vi "纳清DO电极校准.vi"() -> ()   [LabVIEW 2016, in "斯坦道多参数.lvlib"]
uses:
  <vilib>/Utility/miscctls.llb/LVPointTypeDef.ctl
  <vilib>/Analysis/NI_AALBase.lvlib
panel:
  out "滤波设定":dbl
  out "标液2":string="饱和标准液"
  out "标液1":string="零点标准液"
  out "第二点信号值":dbl
  out "第一点信号值":dbl
  out "盐度":sgl format="%#.2f"
  out "大气压力":dbl format="%#.2f"
  out "饱和值":sgl format="%#.2f"
  out "报警信息":string
  out "通讯状态":string
  out "第二点校准值":dbl
  out "第一点校准值":dbl
  in  "校准停止":bool
  in  "校准启动":bool
  in  "校准模式":u16(ring)=1 items=["两点校准", "单点校准"]
  out "最小值":sgl format="%#.2f"
  out "最大值":sgl format="%#.2f"
  out "波形图表":dbl(graph) caption="历史曲线"
  out "mean":dbl caption="均值" format="%#.2f"
  out "standard deviation":dbl caption="标准差" format="%#.2f"
  out "变异系数":dbl format="%#.6f"
  out "测量值":sgl format="%#.2f"
  out "提示":string
  out "原始光强数值":sgl caption="信号值" format="%#.6f"
  out "温度":dbl format="%#.2f"
  # "DO电极设定"
  # "℃"
  # "mg/L"
  # "%"
  # "nA"
  # "kPa"
  # "ppt"
  # "请选择校准模式:"
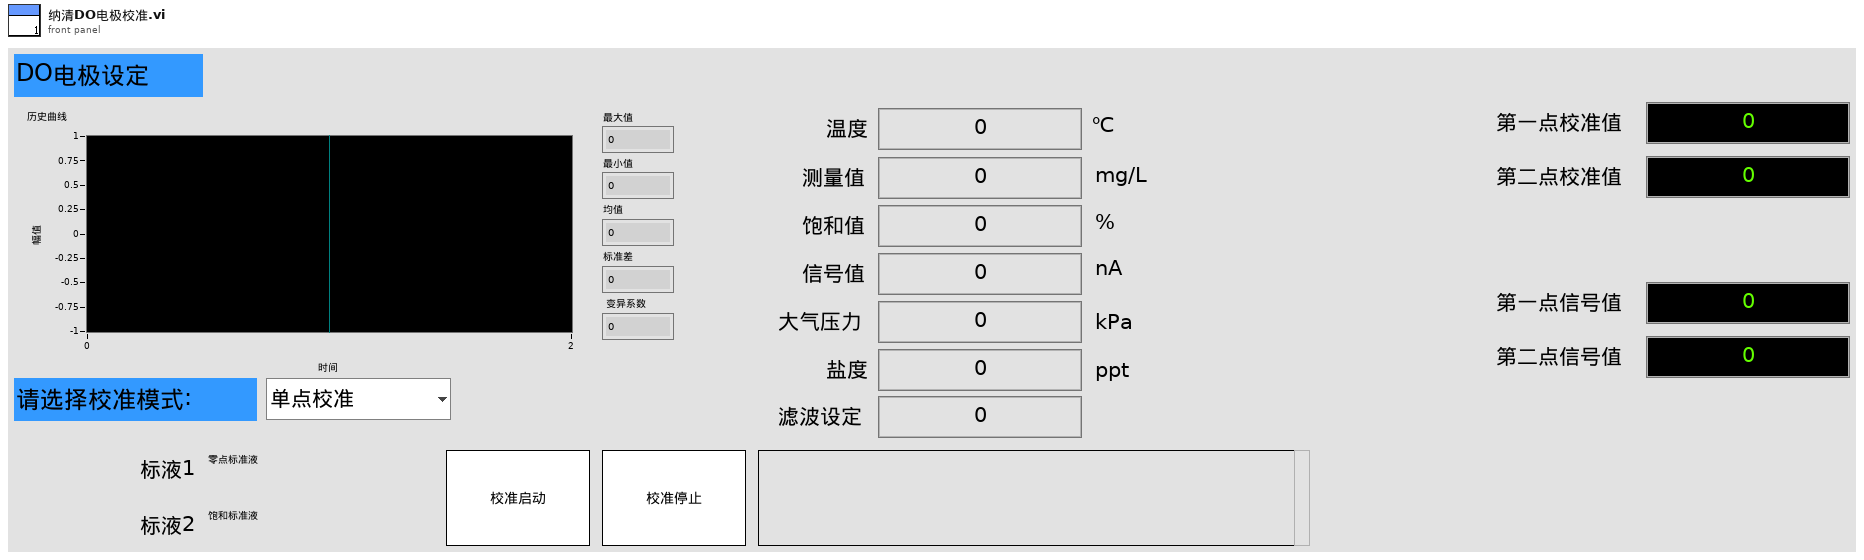
[diagram p1: front panel]
types:
  T1 = enum16{"pH", "DO", "Cond", "Turb", "ORP", "叶绿素a", "藻密度"}
  T2 = typedef "LVPointTypeDef.ctl" = cluster{"Horizontal":i16, "Vertical":i16}
  T3 = cluster{"报警码":u16, "溶解氧数值（mg/L）":sgl, "溶解氧数据（%）":sgl, "温度数据":sgl, "溶解氧原始信号 nA":sgl, "大气压力":sgl, "盐度":sgl, "0X0009_NC":string, "产品名称":string, "序列号":string, "硬件版本":string, "软件版本":string, "通讯地址":u16, "波特率":u16, "设备类型":u16, "0X0026_NC":string, "第一点原始数据":sgl, "第一点校准数据":sgl, "第二点原始数据":sgl, "第二点校准数据":sgl, "探头校准命令":u16, "温度校准参数":sgl, "温度校准命令":u16}
  T4 = cluster{"pH":u32, "DO":u32, "Cond":u32, "Turb":u32, "叶绿素a":u32, "藻密度":u32, "ORP":u32}
  T5 = enum8{"Enabled", "Disabled", "Disabled and Grayed Out"}
  T6 = cluster{"报警码":u16, "溶解氧数值（mg/L）":sgl, "溶解氧数据（%）":sgl, "温度数据":sgl, "溶解氧原始信号 nA":sgl, "大气压力":sgl, "盐度":sgl, "0X0009_NC":string, "产品名称":string, "序列号":string, "硬件版本":string, "软件版本":string, "通讯地址":u16, "波特率":u16, "设备类型":u16, "0X0026_NC":string, "第一点原始数据":sgl, "0X0033 NC":sgl, "第二点原始数据":sgl, "0X0037 NC":sgl, "探头校准命令":u16, "温度校准参数":sgl, "温度校准命令":u16}
  T7 = cluster{"ph":bool, "DO":bool, "Cond":bool, "Turb":bool, "叶绿素a":bool, "藻密度":bool, "ORP":bool}
  T8 = cluster{"温度测量值":sgl, "测量值":sgl, "温度偏移修正值":sgl, "信号值":sgl}
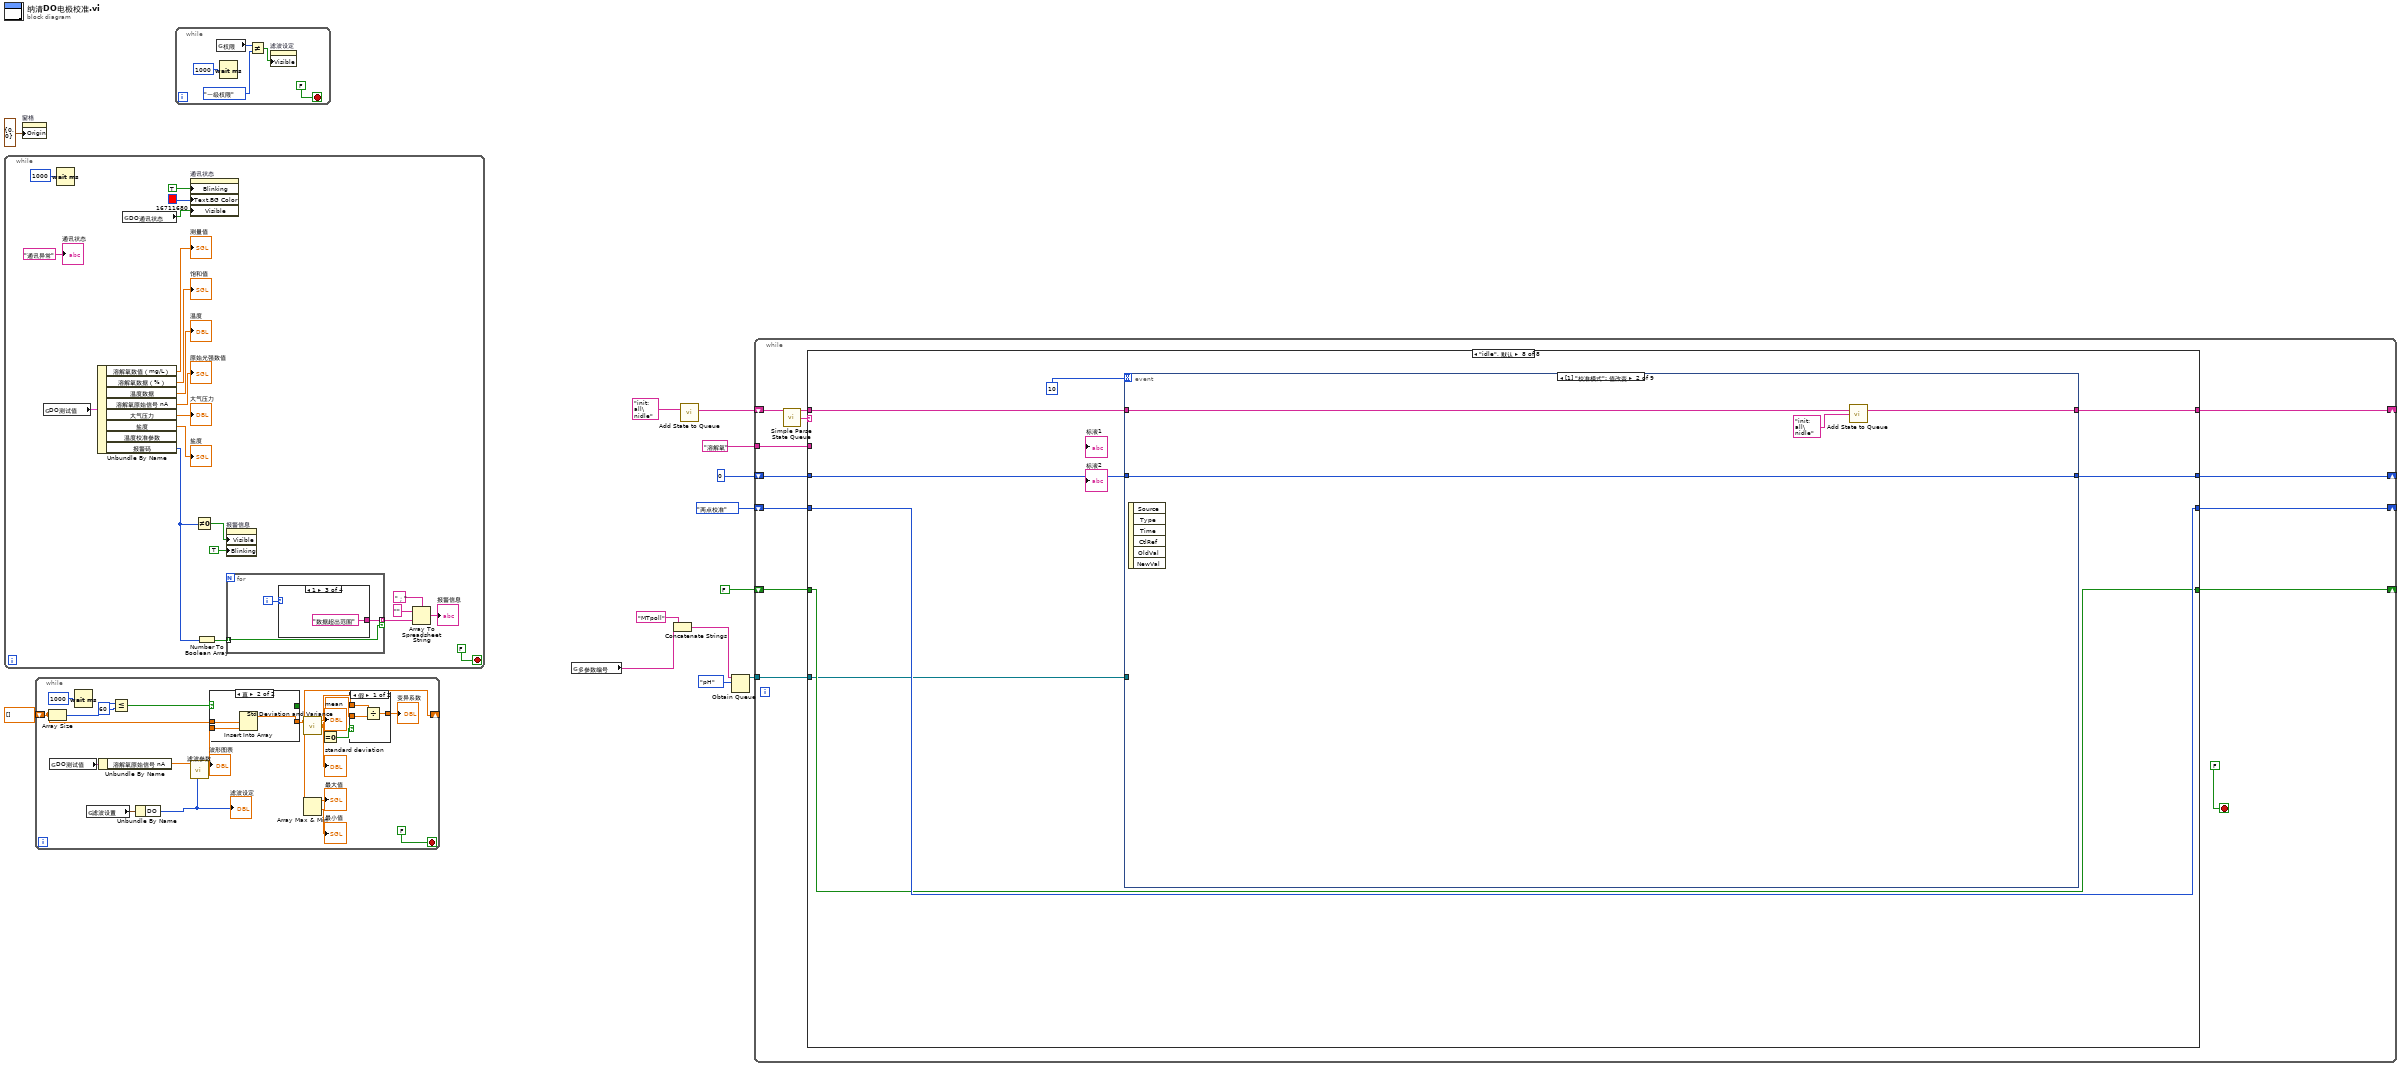
[diagram p0: block diagram]
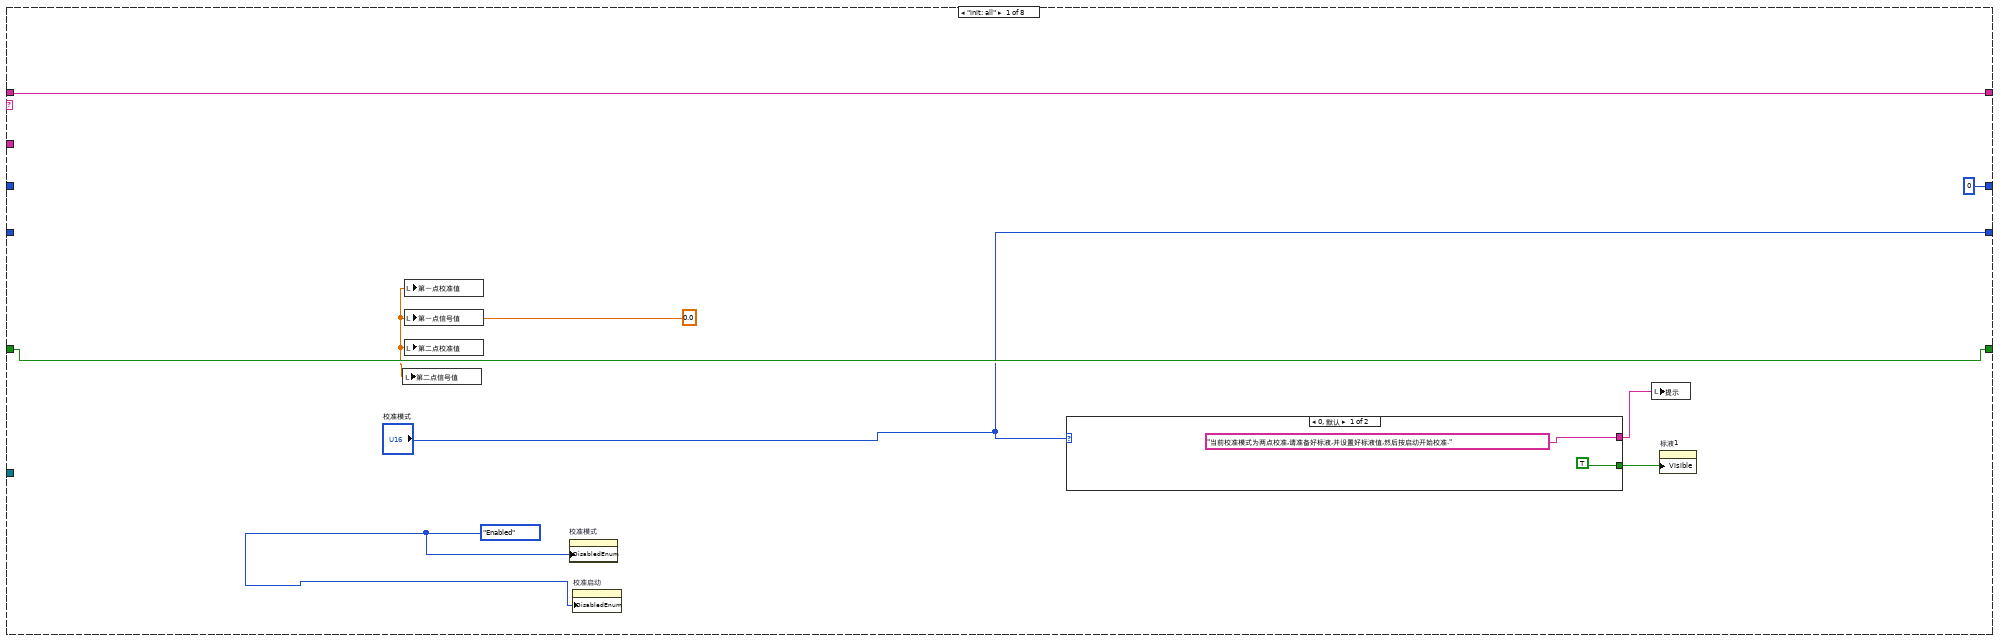
[diagram p2: hidden frame]
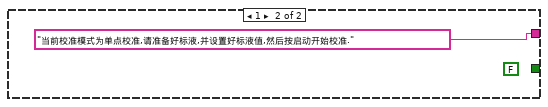
[diagram p3: hidden frame]
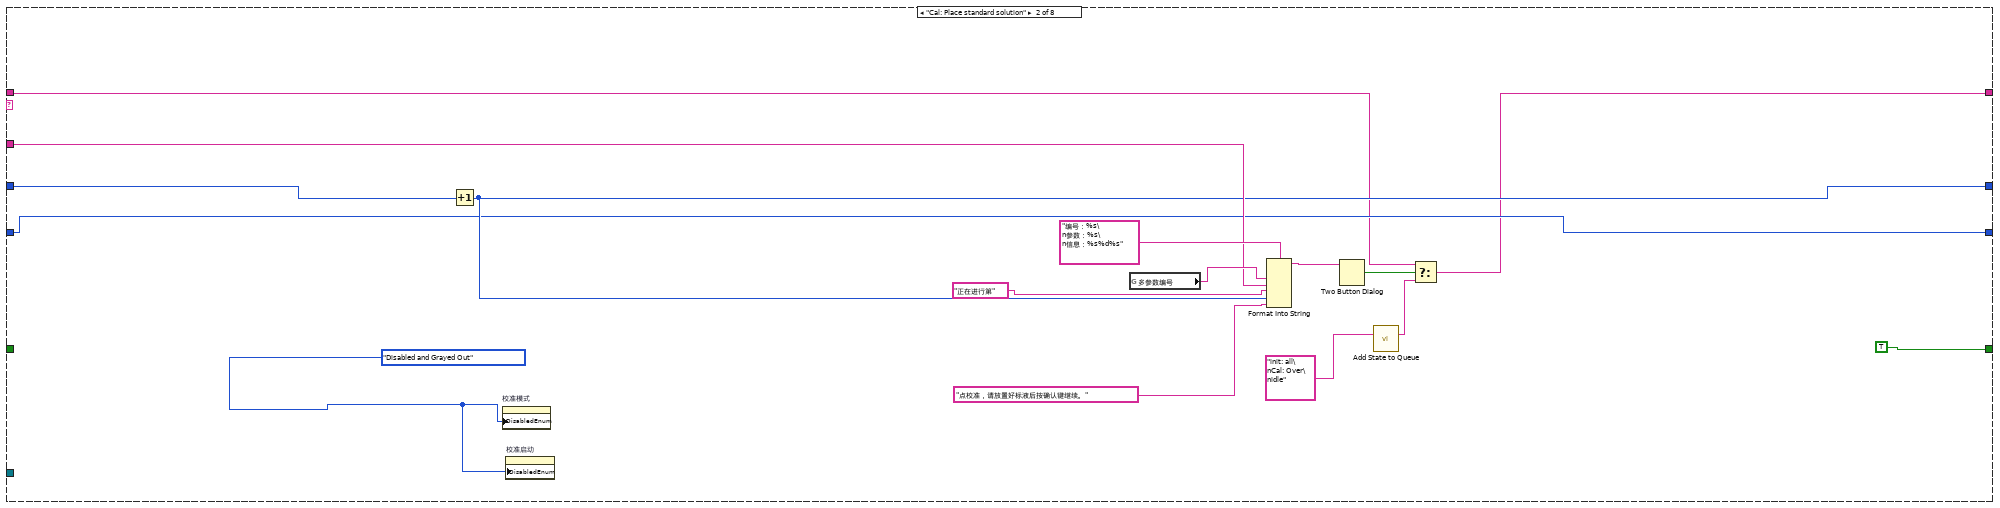
[diagram p4: hidden frame]
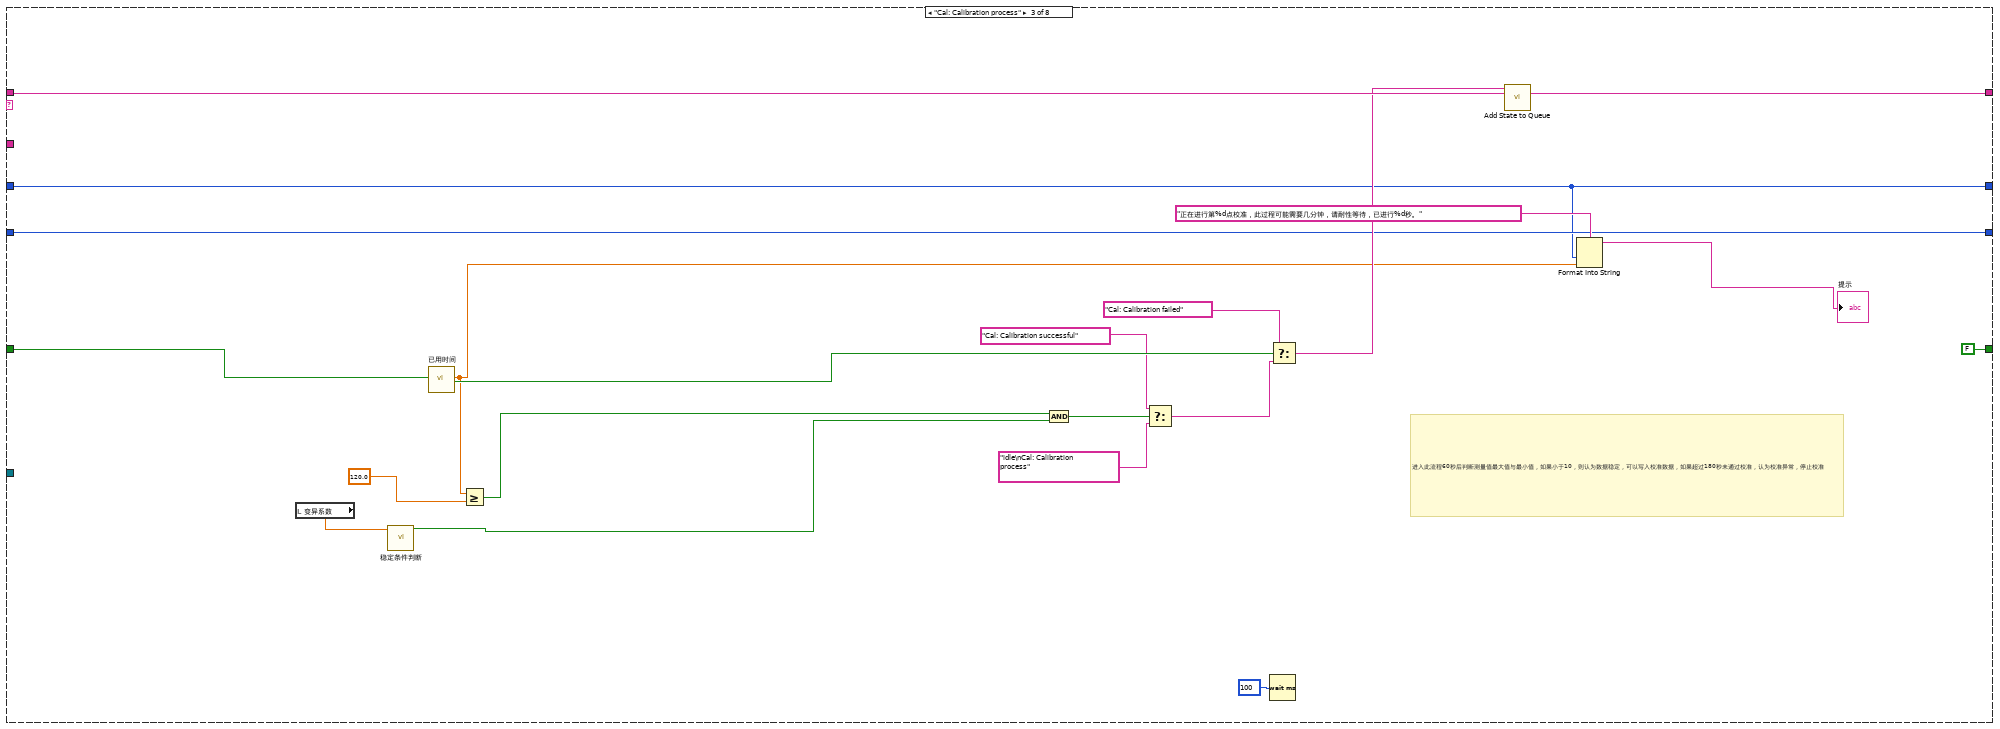
[diagram p5: hidden frame]
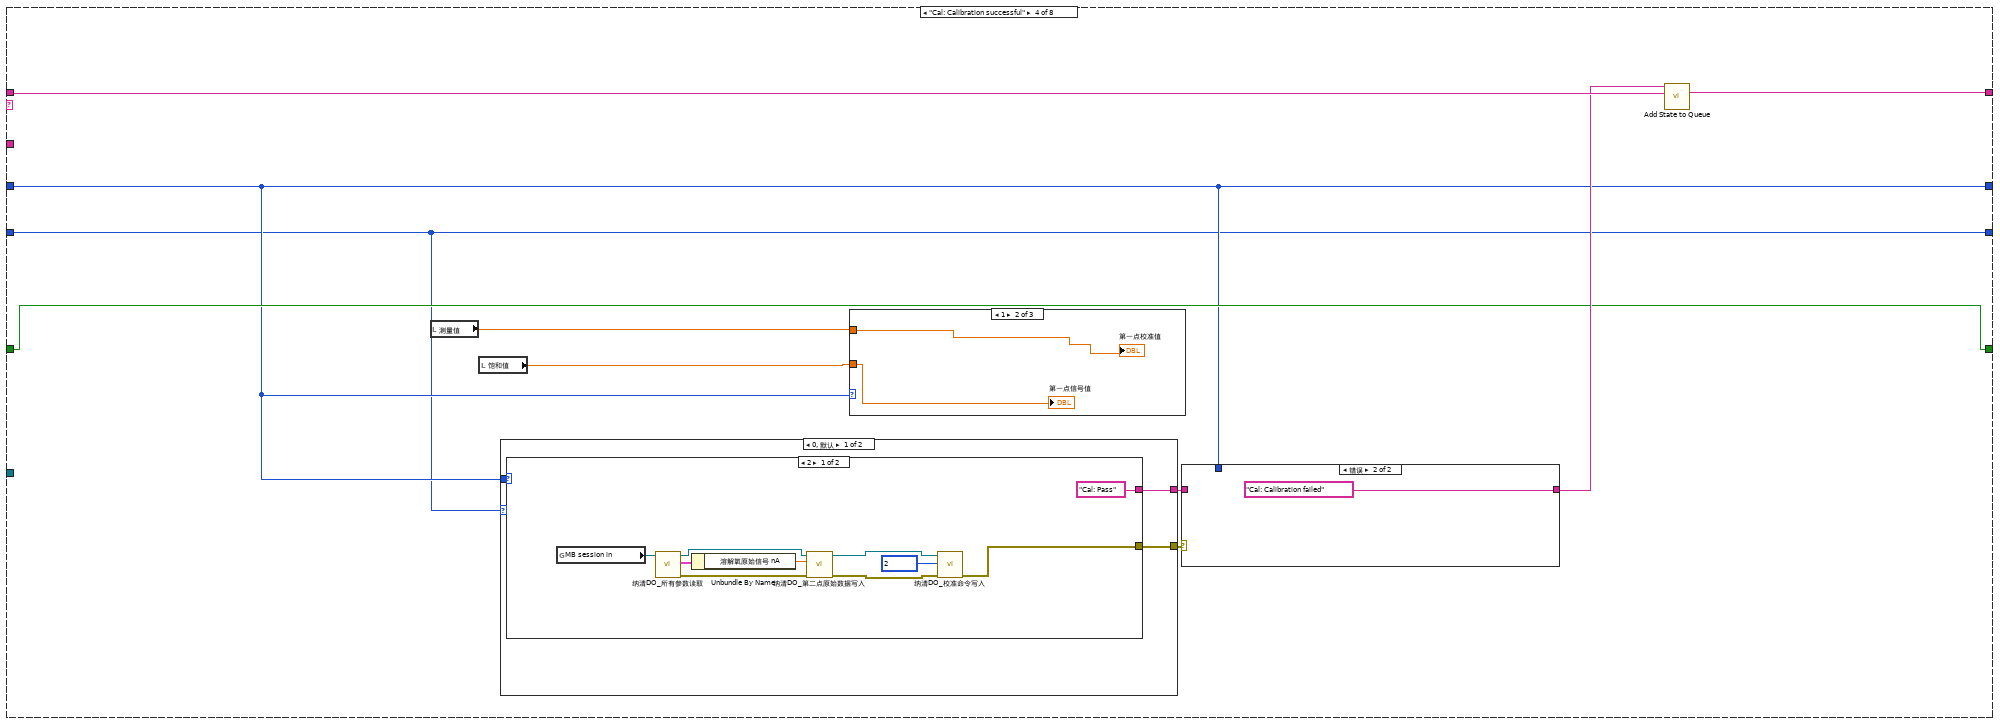
[diagram p6: hidden frame]
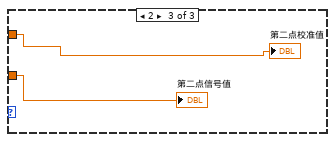
[diagram p8: hidden frame]
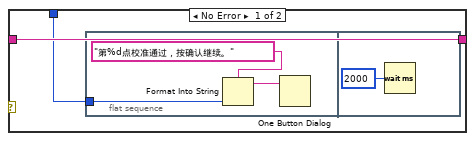
[diagram p9: hidden frame]
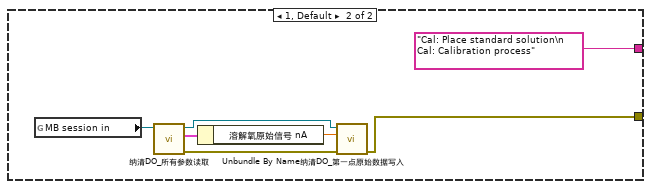
[diagram p10: hidden frame]
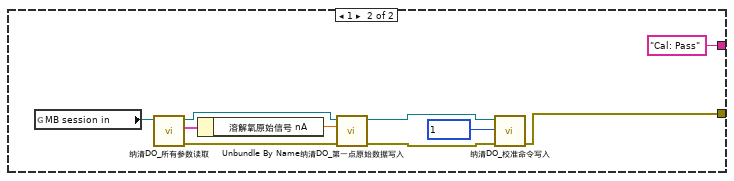
[diagram p11: hidden frame]
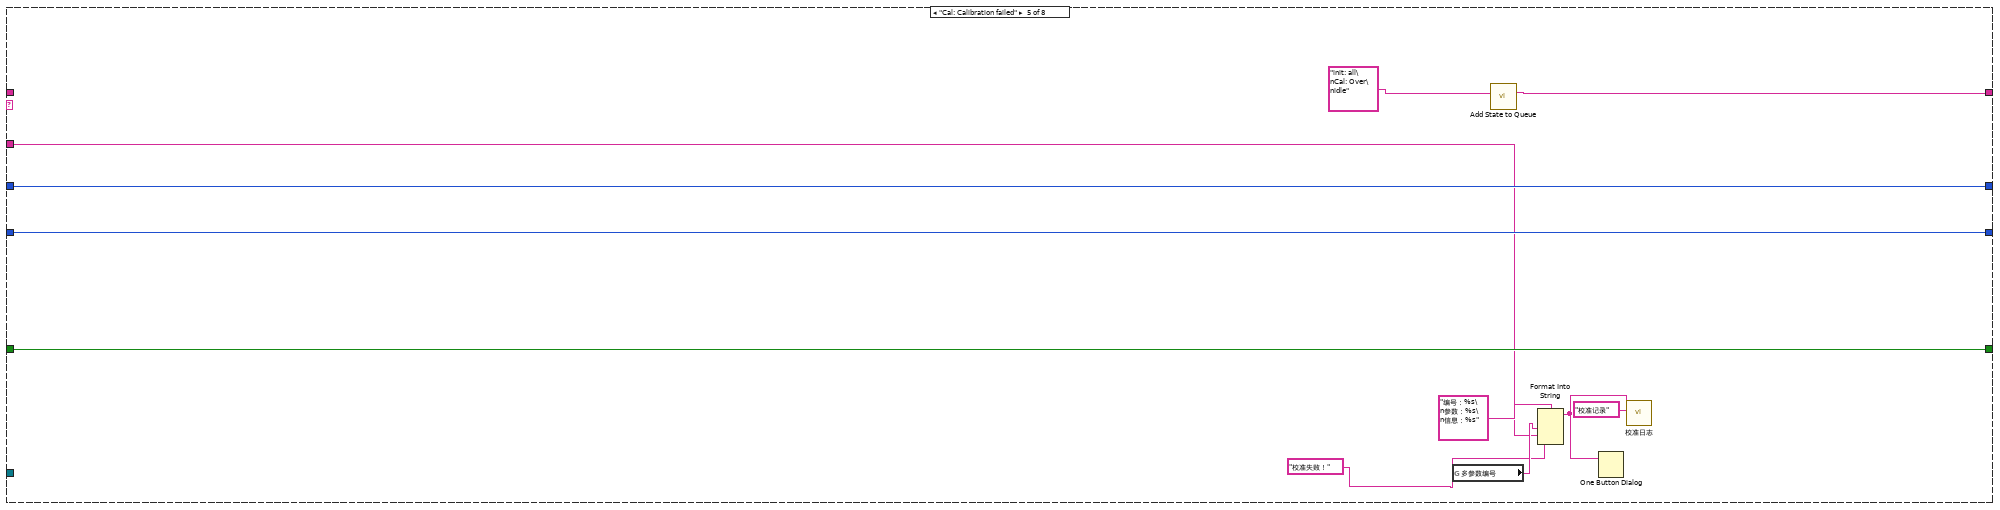
[diagram p12: hidden frame]
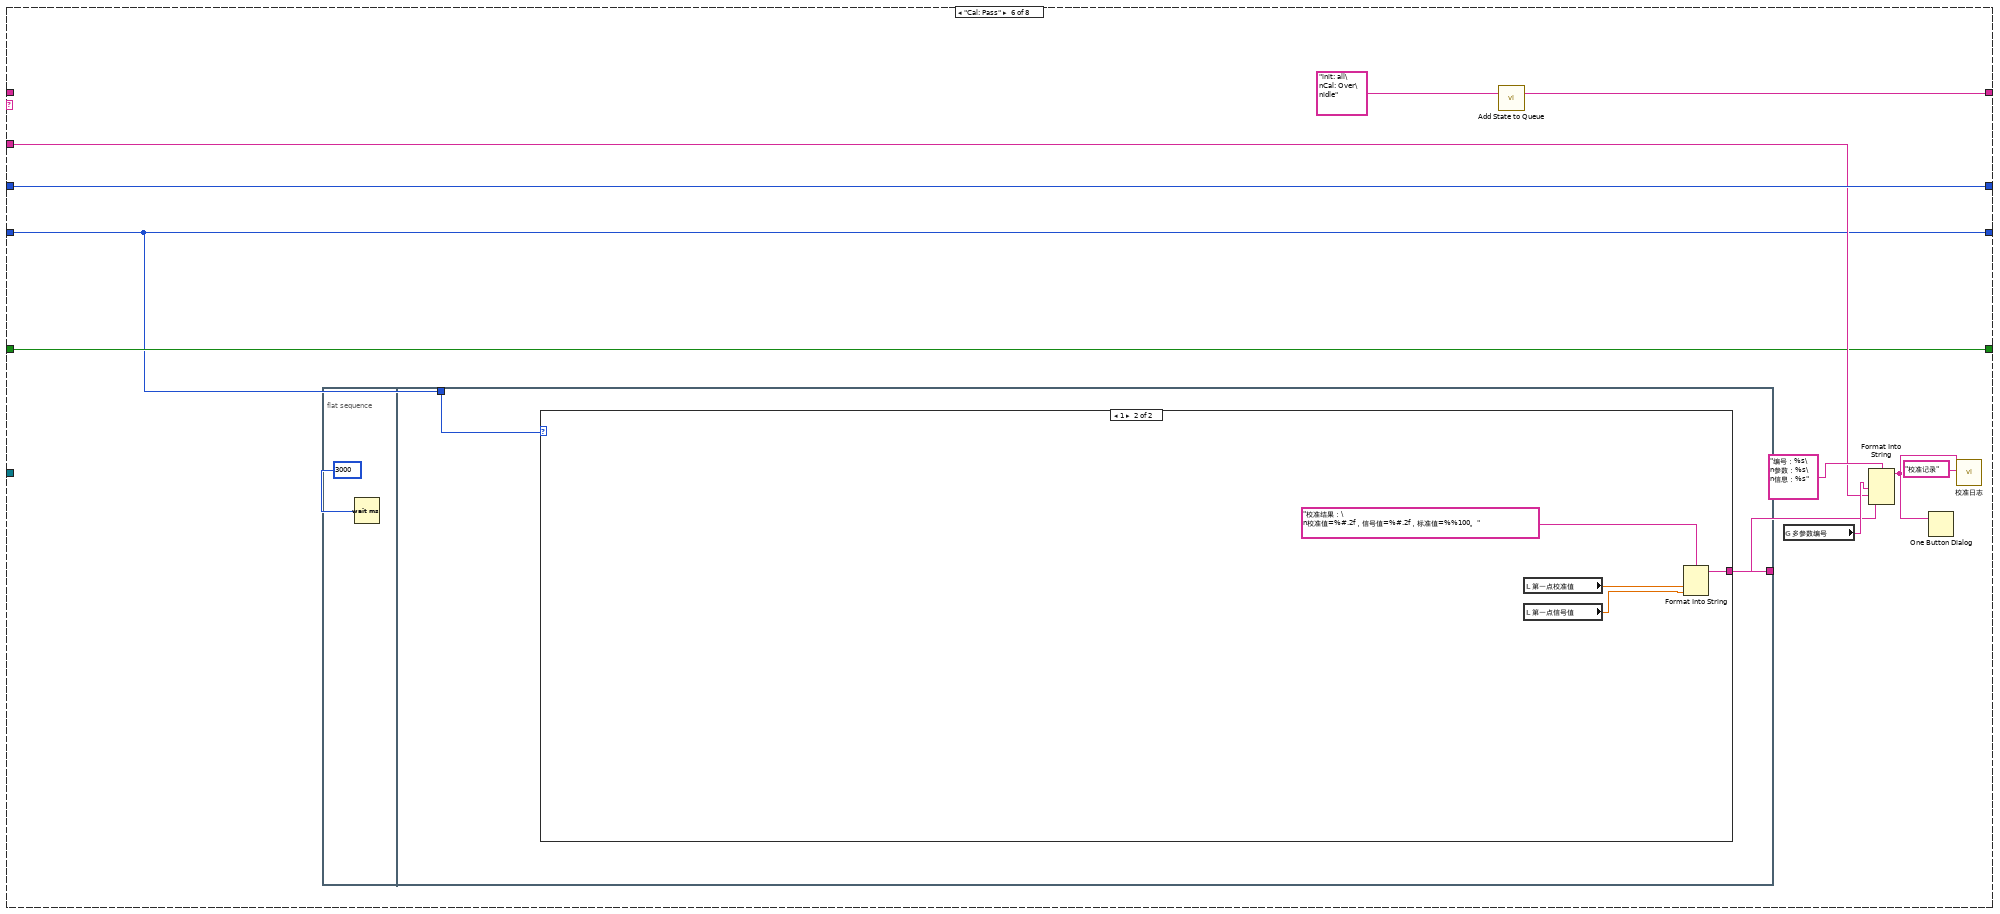
[diagram p13: hidden frame]
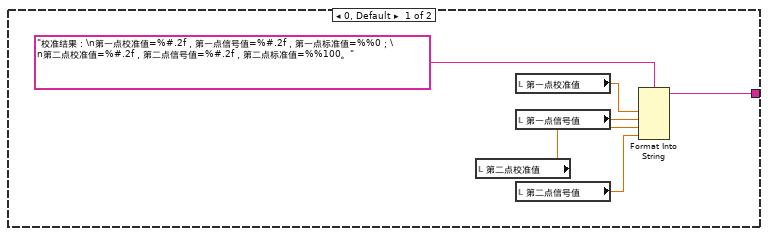
[diagram p14: hidden frame]
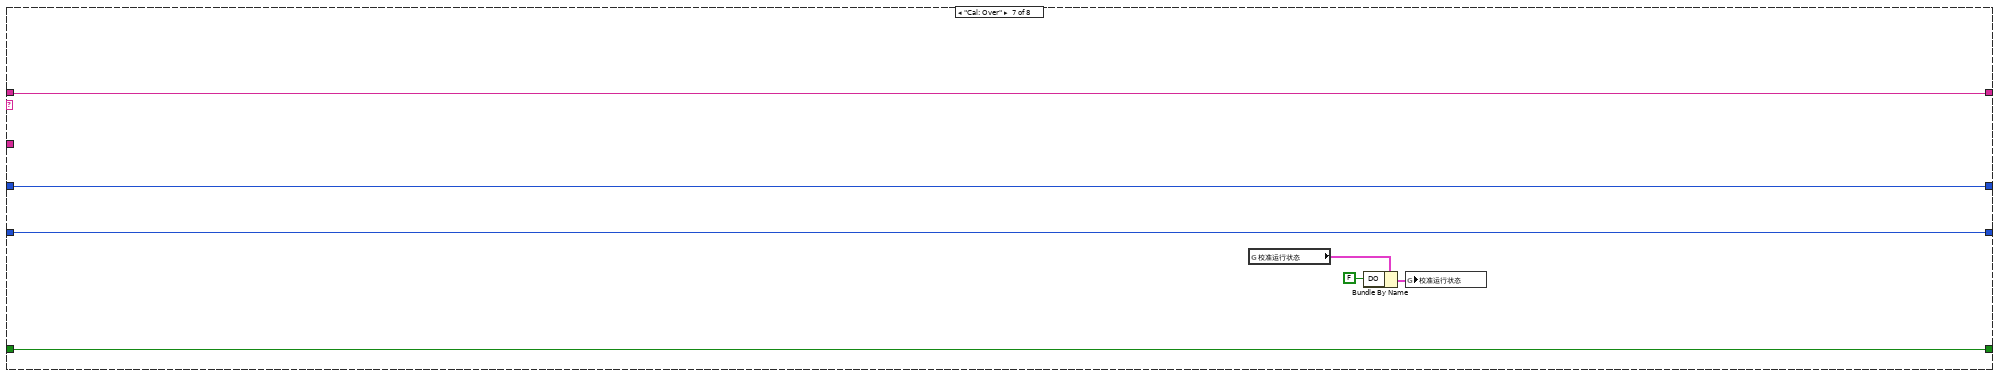
[diagram p15: hidden frame]
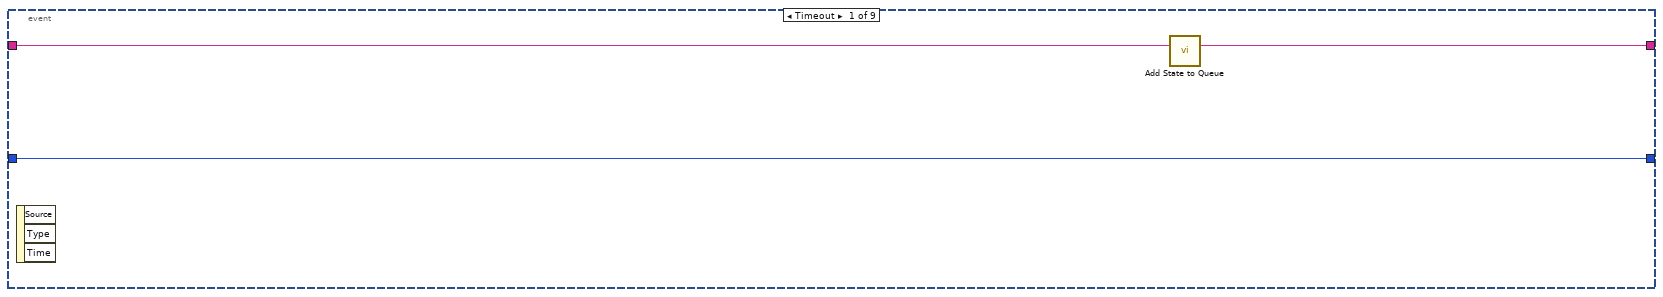
[diagram p16: hidden frame]
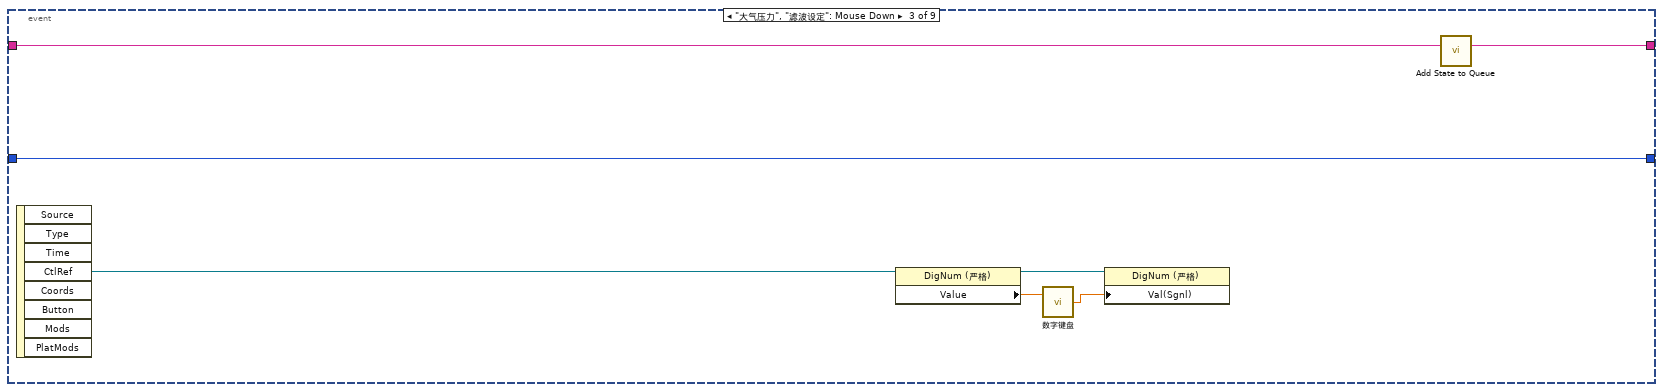
[diagram p17: hidden frame]
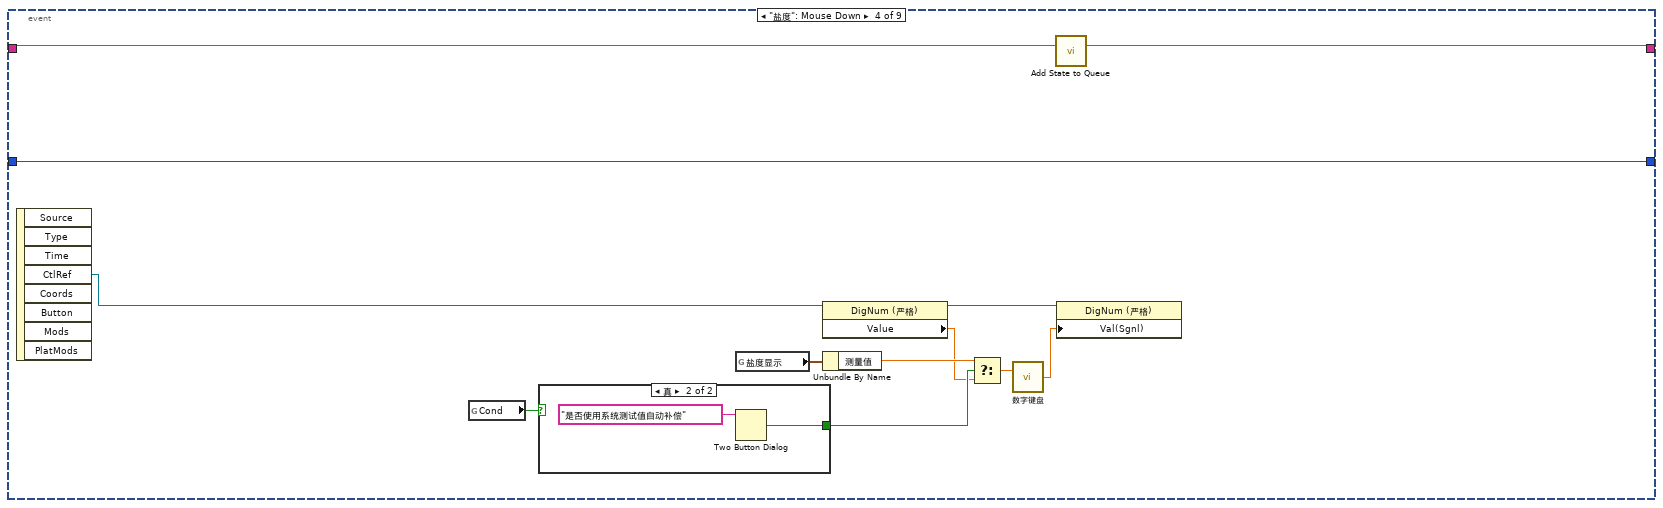
[diagram p18: hidden frame]
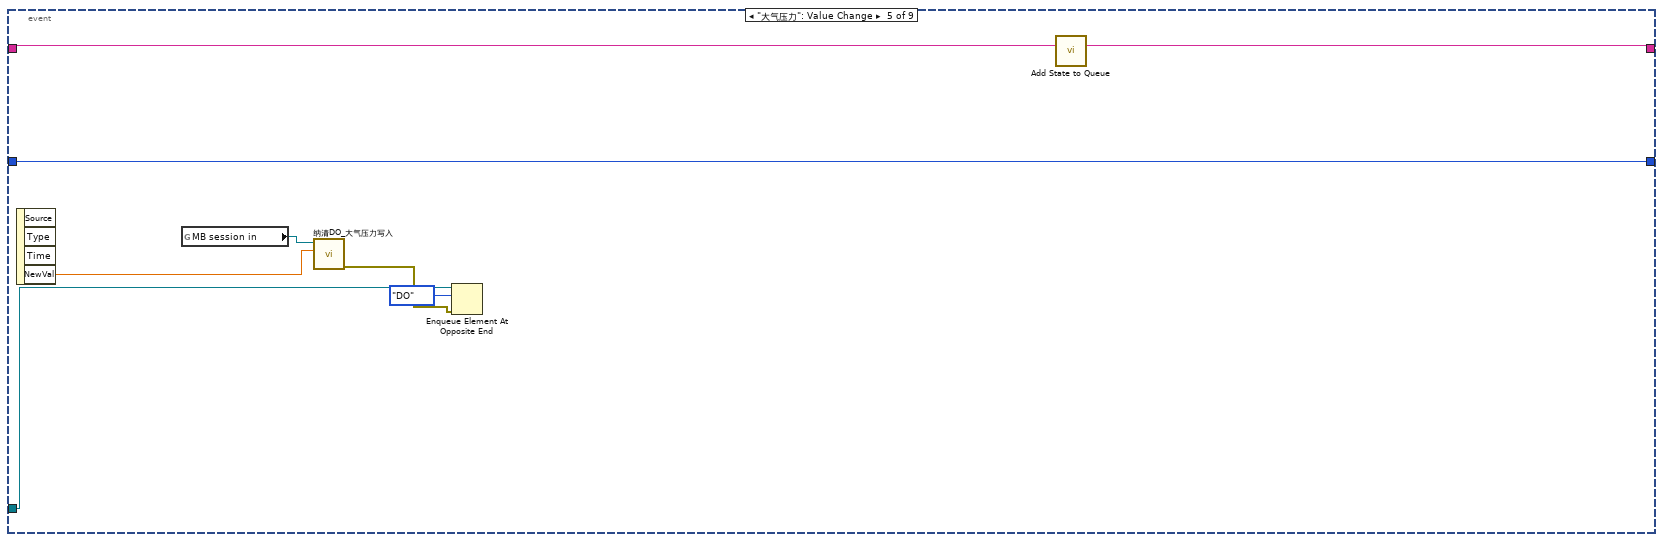
[diagram p20: hidden frame]
diagram:
  n1 = while {
    stop <- FALSE stop-if-true
    n2 = global read "纳清过程全局变量.vi" "DO测试值"() -> (w32:T3)
    n3 = Wait (ms)(milliseconds to wait=u32 1000 ("等待时间（毫秒）")) -> ()  [unwired: 1 out]
    n4 = Unbundle By Name(w32) -> ("溶解氧数值（mg/L）"=→"测量值":sgl, "溶解氧数据（%）"=→"饱和值":sgl, "温度数据"=→"温度":sgl, "溶解氧原始信号 nA"=→"原始光强数值":sgl, "大气压力"=→"大气压力":sgl, "盐度"=→"盐度":sgl, "报警码"=w19:u16)  [unwired: 1 out]
    n5 = global read "多参数全局变量.vi" "DO通讯状态"() -> (w25:bool)
    n6 = property on="通讯状态" class="Str"("Blinking"=TRUE ("闪烁"), "Text.BG Color"=u32 16711680, "Visible"=w25) -> ()  [unwired: 2 in, 2 out]
    n7 = Not Equal To 0?(x=w19) -> (x != 0?=w18:bool)
    n8 = Number To Boolean Array(number=w19) -> (Boolean array=w24:bool[])
    n9 = property on="报警信息" class="Str"("Visible"=w18, "Blinking"=TRUE ("闪烁")) -> ()  [unwired: 2 in, 2 out]
    n10 = for {
      tunnel: w24 -> [w35] mode=indexing
      tunnel: [w36] -> w23 mode=indexing if=w35
      i -> [w37]
      n11 = case shown="1" w37 {
        tunnel: [_ "温度超出范围" "数据超出范围" "温度传感器故障"] -> w36
        frame Default {
        }
        frame 0 {
        }
        frame 1 {
        }
        frame 8 {
        }
      }
    }
    n12 = Array To Spreadsheet String(delimiter (Tab)="；" ("分隔符(Tab)"), array=w23, 3:"" ("格式字符串")) -> (spreadsheet string=→"报警信息":string)
    "通讯状态" <- "通讯异常" ("当前串口")
  }
  n13 = property on="窗格" class="Pane"("Origin"=T2 {"Horizontal"=0, "Vertical"=0} ("原点")) -> ()  [unwired: 2 in, 2 out]
  n14 = while {
    shift-right: [w48] -> _
    shift-left: sgl[] [] -> [w54]
    stop <- FALSE stop-if-true
    n15 = Array Size(array=w54) -> (size(s)=w56:i32)
    n16 = global read "纳清过程全局变量.vi" "DO测试值"() -> (w45:T3)
    n17 = Wait (ms)(milliseconds to wait=u32 1000 ("等待时间（毫秒）")) -> ()  [unwired: 1 out]
    n18 = global read "断电保存变量.vi" "滤波设置"() -> (w42:T4)
    n19 = Unbundle By Name(w45) -> ("溶解氧原始信号 nA"=w44:sgl)
    n20 = Less Or Equal?(x=w56, y=60) -> (x <= y?=w55:bool)
    n21 = Unbundle By Name(w42) -> ("DO"=w41:u32)
    "滤波设定" <- w41
    n22 = call "滤波参数.vi"("滤波次数"=w41, "x"=w44) -> ("mode"=w43:dbl)  [unwired: 9 in]
    "波形图表" <- w43
    n23 = case shown="真" w55 {
      tunnel: w54 -> [w67 w70]
      tunnel: w43 -> [w65 w69]
      tunnel: [w63 w68] -> w48
      tunnel: [TRUE _] -> _
      frame False {
        n24 = Replace Array Subset(array=w67, new element=w65) -> (w66:sgl[])  [unwired: 1 in]
        n25 = Rotate 1D Array(1:w66, 2:-1 ("n")) -> (0:w63:sgl[])
      }
      frame True {
        n26 = Insert Into Array(array=w70, new element=w69) -> (w68:sgl[])  [unwired: 1 in]
      }
    }
    n27 = call <vilib>:"Std Deviation and Variance.vi"("X"=w48) -> ("mean"=w52:dbl, "standard deviation"=w51:dbl)  [unwired: 1 in, 1 out]
    "mean" <- w52
    "standard deviation" <- w51
    n28 = Array Max & Min(array=w48) -> (max value=→"最大值":sgl, min value=→"最小值":sgl)  [unwired: 2 out]
    n29 = Equal To 0?(x=w52) -> (x = 0?=w53:bool)
    n30 = case shown="假" w53 {
      tunnel: w51 -> [w61 _]
      tunnel: [w60 _] -> w50
      tunnel: w52 -> [w59 _]
      frame False {
        n31 = Divide(x=w61, y=w59) -> (x/y=w60:dbl)
      }
      frame True {
      }
    }
    "变异系数" <- w50
  }
  n32 = while {
    stop <- FALSE stop-if-true
    n33 = global read "多参数全局变量.vi" "权限"() -> (w74:enum16{"一级权限", "二级权限", "三级权限"})
    n34 = Wait (ms)(milliseconds to wait=u32 1000 ("等待时间（毫秒）")) -> ()  [unwired: 1 out]
    n35 = Not Equal?(x=w74, y=enum16{"一级权限", "二级权限", "三级权限"}."一级权限") -> (x != y?=w71:bool)
    n36 = property on="滤波设定" class="DigNum (严格)"("Visible"=w71) -> ()  [unwired: 2 in, 2 out]
  }
  n37 = global read "多参数全局变量.vi" "多参数编号"() -> (w2:string)
  n38 = Concatenate Strings("MTpoll" ("名称（未命名）"), w2) -> (w4:string)
  n39 = call "Add State to Queue.vi"("State(s) In (\"\")"="init: all\nidle" ("State(s) In (\"\")")) -> ("States Out"=w10:string)  [unwired: 14 in]
  n40 = Obtain Queue(name (unnamed)=w4, element data type=T1."pH" ("枚举")) -> (queue out=w1:refnum<queue>)  [unwired: 3 in, 2 out]
  n41 = while {
    shift-right: [w84] -> _
    shift-left: w10 -> [w88]
    shift-right: [w81] -> _
    shift-left: 0 -> [w83]
    tunnel: "溶解氧" ("State(s) In (\"\")") -> [w82]
    shift-right: [w79] -> _
    shift-left: enum16{"两点校准", "单点校准"}."两点校准" ("校准模式") -> [w80]
    shift-right: [w77] -> _
    shift-left: FALSE -> [w78]
    tunnel: w1 -> [w76]
    stop <- FALSE stop-if-true
    n42 = call "Simple Parse State Queue.vi"("State Queue"=w88) -> ("Remain States"=w85:string, "Next State"=w86:string)  [unwired: 13 in]
    n43 = case shown="\"idle\", 默认" w86 {
      tunnel: w85 -> [w96 w103 w135 w144 _ _ w229 w237]
      tunnel: [w96 w102 w134 w143 w195 w200 w229 w236] -> w84
      tunnel: w83 -> [_ w111 w120 w138 w198 w209 w228 w234]
      tunnel: w82 -> [_ w112 _ _ w189 w205 _ _]
      tunnel: [0 w109 w120 w138 w198 w209 w228 w235] -> w81
      tunnel: w80 -> [_ w108 w121 w137 w197 w201 w227 w233]
      tunnel: ["校准模式" w108 w121 w137 w197 w201 w227 w233] -> w79
      tunnel: w78 -> [w93 _ w123 w139 w196 w204 w226 w231]
      tunnel: [w93 TRUE FALSE w139 w196 w204 w226 w231] -> w77
      tunnel: w76 -> [_ _ _ _ _ _ _ w230]
      frame "init: all" {
        w90 = T5."Enabled" ("禁用")
        w92 = 0.0 ("第一点校准值")
        n44 = local write "第二点信号值"(w92) -> ()
        n45 = local write "第一点校准值"(w92) -> ()
        n46 = local write "第一点信号值"(w92) -> ()
        n47 = local write "第二点校准值"(w92) -> ()
        n48 = property on="校准模式" class="Ring (严格)"("DisabledEnum"=w90) -> ()  [unwired: 2 in, 2 out]
        n49 = property on="校准启动" class="Bool"("DisabledEnum"=w90) -> ()  [unwired: 2 in, 2 out]
        n50 = case shown="0, 默认" "校准模式" {
          tunnel: ["当前校准模式为两点校准,请准备好标液,并设置好标液值,然后按启动开始校准." ("提示") "当前校准模式为单点校准,请准备好标液,并设置好标液值,然后按启动开始校准." ("提示")] -> w95
          tunnel: [TRUE ("可见") _] -> w89
          frame 0, Default {
          }
          frame 1 {
            (unwired) FALSE ("可见")
          }
        }
        n51 = local write "提示"(w95) -> ()
        n52 = property on="标液1" class="Str"("Visible"=w89) -> ()  [unwired: 2 in, 2 out]
      }
      frame "Cal: Place standard solution" {
        w101 = T5."Disabled and Grayed Out" ("禁用")
        n53 = Increment(x=w111) -> (x+1=w109:i32)
        n54 = property on="校准模式" class="Ring (严格)"("DisabledEnum"=w101) -> ()  [unwired: 2 in, 2 out]
        n55 = property on="校准启动" class="Bool"("DisabledEnum"=w101) -> ()  [unwired: 2 in, 2 out]
        n56 = global read "多参数全局变量.vi" "多参数编号"() -> (w114:string)
        n57 = Format Into String(format string="编号：%s\n参数：%s\n信息：%s%d%s" ("格式字符串"), w114, w112, "正在进行第" ("消息"), w109, "点校准，请放置好标液后按确认键继续。" ("消息")) -> (resulting string=w106:string)  [unwired: 2 in, 1 out]
        n58 = Two Button Dialog(message=w106) -> (T button?=w105:bool)  [unwired: 2 in]
        n59 = call "Add State to Queue.vi"("State(s) In (\"\")"="init: all\nCal: Over\nidle" ("State(s) In (\"\")")) -> ("States Out"=w104:string)  [unwired: 14 in]
        n60 = Select(t=w103, s=w105, f=w104) -> (s? t:f=w102:string)
      }
      frame "Cal: Calibration process" {
        # "进入此流程60秒后判断测量值最大值与最小值，如果小于10，则认为数据稳定，可以写入校准数据，如果超过180秒未通过校准，认为校准异常，停止校准"
        n61 = local read "变异系数"() -> (w117:dbl)
        n62 = call "稳定条件判断.vi"("变异系数"=w117) -> ("布尔"=w116:bool)  [unwired: 10 in]
        n63 = call "已用时间"("Reset"=w123) -> ("Elapsed Time (s)"=w119:dbl, "Time has Elapsed"=w136:bool)  [unwired: 11 in, 6 out]
        n64 = Greater Or Equal?(x=w119, y=120.0) -> (x >= y?=w131:bool)
        n65 = And(x=w131, y=w116) -> (x .and. y?=w128:bool)
        n66 = Select(t="Cal: Calibration successful" ("State(s) In (\"\")"), s=w128, f="idle\nCal: Calibration process" ("State(s) In (\"\")")) -> (s? t:f=w127:string)
        n67 = Wait (ms)(milliseconds to wait=u32 100 ("等待时间（毫秒）")) -> ()  [unwired: 1 out]
        n68 = Select(t="Cal: Calibration failed" ("State(s) In (\"\")"), s=w136, f=w127) -> (s? t:f=w126:string)
        n69 = call "Add State to Queue.vi"("State(s) In Front (\"\")"=w126, "State(s) In (\"\")"=w135) -> ("States Out"=w134:string)  [unwired: 13 in]
        n70 = Format Into String(format string="正在进行第%d点校准，此过程可能需要几分钟，请耐性等待，已进行%d秒。" ("格式字符串"), w120, w119) -> (resulting string=→"提示":string)  [unwired: 2 in, 1 out]
      }
      frame "Cal: Calibration successful" {
        n71 = local read "测量值"() -> (w140:sgl)
        n72 = local read "饱和值"() -> (w141:sgl)
        n73 = case shown="0, 默认" w137 {
          tunnel: [w160 w178] -> w146
          tunnel: [w159 "Cal: Pass" ("State(s) In (\"\")")] -> w145
          tunnel: w138 -> [w158 _]
          frame 0, Default {
            n74 = case shown="2" w158 {
              tunnel: [w162 w171] -> w160
              tunnel: ["Cal: Pass" ("State(s) In (\"\")") "Cal: Place standard solution\n Cal: Calibration process" ("State(s) In (\"\")")] -> w159
              frame 2 {
                n75 = global read "多参数全局变量.vi" "MB session in"() -> (w167:refnum<class "MB_Master.lvclass">)
                n76 = call "纳清DO_所有参数读取.vi"("MB session in"=w167) -> ("error out"=w169:errorcluster, "输出值"=w166:T6, "MB session out"=w168:refnum<class "MB_Master.lvclass">)  [unwired: 8 in]
                n77 = Unbundle By Name(w166) -> ("溶解氧原始信号 nA"=w165:sgl)
                n78 = call "纳清DO_第二点原始数据写入.vi"("error in (no error)"=w169, "数值"=w165, "MB session in"=w168) -> ("error out"=w164:errorcluster, "MB session out"=w163:refnum<class "MB_Master.lvclass">)  [unwired: 7 in]
                n79 = call "纳清DO_校准命令写入.vi"("error in (no error)"=w164, "数值"=u16 2 ("starting address"), "MB session in"=w163) -> ("error out"=w162:errorcluster)  [unwired: 7 in, 1 out]
              }
              frame 1, Default {
                n80 = global read "多参数全局变量.vi" "MB session in"() -> (w174:refnum<class "MB_Master.lvclass">)
                n81 = call "纳清DO_所有参数读取.vi"("MB session in"=w174) -> ("error out"=w176:errorcluster, "输出值"=w173:T6, "MB session out"=w175:refnum<class "MB_Master.lvclass">)  [unwired: 8 in]
                n82 = Unbundle By Name(w173) -> ("溶解氧原始信号 nA"=w172:sgl)
                n83 = call "纳清DO_第一点原始数据写入.vi"("error in (no error)"=w176, "数值"=w172, "MB session in"=w175) -> ("error out"=w171:errorcluster)  [unwired: 7 in, 1 out]
              }
            }
          }
          frame 1 {
            n84 = global read "多参数全局变量.vi" "MB session in"() -> (w184:refnum<class "MB_Master.lvclass">)
            n85 = call "纳清DO_所有参数读取.vi"("MB session in"=w184) -> ("error out"=w186:errorcluster, "输出值"=w183:T6, "MB session out"=w185:refnum<class "MB_Master.lvclass">)  [unwired: 8 in]
            n86 = Unbundle By Name(w183) -> ("溶解氧原始信号 nA"=w182:sgl)
            n87 = call "纳清DO_第一点原始数据写入.vi"("error in (no error)"=w186, "数值"=w182, "MB session in"=w185) -> ("error out"=w181:errorcluster, "MB session out"=w180:refnum<class "MB_Master.lvclass">)  [unwired: 7 in]
            n88 = call "纳清DO_校准命令写入.vi"("error in (no error)"=w181, "数值"=u16 1 ("starting address"), "MB session in"=w180) -> ("error out"=w178:errorcluster)  [unwired: 7 in, 1 out]
          }
        }
        n89 = case shown="1" w138 {
          tunnel: w141 -> [_ w148 w150]
          tunnel: w140 -> [_ w147 w149]
          frame 0, Default {
          }
          frame 1 {
            "第一点信号值" <- w148
            "第一点校准值" <- w147
          }
          frame 2 {
            "第二点信号值" <- w150
            "第二点校准值" <- w149
          }
        }
        n90 = case shown="错误" w146 {
          tunnel: w145 -> [w152 _]
          tunnel: [w152 "Cal: Calibration failed" ("State(s) In (\"\")")] -> w142
          tunnel: w138 -> [w151 _]
          frame No Error {
            n91 = flat-sequence {
              tunnel: w151 -> [w153]
              frame #0 {
                n92 = Format Into String(format string="第%d点校准通过，按确认继续。" ("格式字符串"), w153) -> (resulting string=w155:string)  [unwired: 2 in, 1 out]
                n93 = One Button Dialog(message=w155) -> ()  [unwired: 1 in, 1 out]
              }
              frame #1 {
                n94 = Wait (ms)(milliseconds to wait=u32 2000 ("等待时间（毫秒）")) -> ()  [unwired: 1 out]
              }
            }
          }
          frame Error {
          }
        }
        n95 = call "Add State to Queue.vi"("State(s) In Front (\"\")"=w142, "State(s) In (\"\")"=w144) -> ("States Out"=w143:string)  [unwired: 13 in]
      }
      frame "Cal: Calibration failed" {
        n96 = global read "多参数全局变量.vi" "多参数编号"() -> (w192:string)
        n97 = call "Add State to Queue.vi"("State(s) In (\"\")"="init: all\nCal: Over\nidle" ("State(s) In (\"\")")) -> ("States Out"=w195:string)  [unwired: 14 in]
        n98 = Format Into String(format string="编号：%s\n参数：%s\n信息：%s" ("格式字符串"), w192, w189, "校准失败！" ("消息")) -> (resulting string=w191:string)  [unwired: 2 in, 1 out]
        n99 = One Button Dialog(message=w191) -> ()  [unwired: 1 in, 1 out]
        n100 = call "校准日志.vi"("table"="校准记录", "日志信息"=w191) -> ()  [unwired: 9 in, 1 out]
      }
      frame "Cal: Pass" {
        n101 = flat-sequence {
          tunnel: [w212] -> w202
          tunnel: w201 -> [w211]
          frame #0 {
            n102 = Wait (ms)(milliseconds to wait=u32 3000 ("等待时间（毫秒）")) -> ()  [unwired: 1 out]
          }
          frame #1 {
            n103 = case shown="1" w211 {
              tunnel: [w218 w222] -> w212
              frame 0, Default {
                n104 = local read "第二点校准值"() -> (w214:dbl)
                n105 = local read "第一点校准值"() -> (w216:dbl)
                n106 = local read "第一点信号值"() -> (w217:dbl)
                n107 = local read "第二点信号值"() -> (w213:dbl)
                n108 = Format Into String(format string="校准结果：\n第一点校准值=%#.2f，第一点信号值=%#.2f，第一点标准值=%%0；\n第二点校准值=%#.2f，第二点信号值=%#.2f，第二点标准值=%%100。" ("提示"), w216, w217, w214, w213) -> (resulting string=w218:string)  [unwired: 2 in, 1 out]
              }
              frame 1 {
                n109 = local read "第一点校准值"() -> (w221:dbl)
                n110 = local read "第一点信号值"() -> (w219:dbl)
                n111 = Format Into String(format string="校准结果：\n校准值=%#.2f，信号值=%#.2f，标准值=%%100。" ("提示"), w221, w219) -> (resulting string=w222:string)  [unwired: 2 in, 1 out]
              }
            }
          }
        }
        n112 = call "Add State to Queue.vi"("State(s) In (\"\")"="init: all\nCal: Over\nidle" ("State(s) In (\"\")")) -> ("States Out"=w200:string)  [unwired: 14 in]
        n113 = global read "多参数全局变量.vi" "多参数编号"() -> (w206:string)
        n114 = Format Into String(format string="编号：%s\n参数：%s\n信息：%s" ("格式字符串"), w206, w205, w202) -> (resulting string=w203:string)  [unwired: 2 in, 1 out]
        n115 = One Button Dialog(message=w203) -> ()  [unwired: 1 in, 1 out]
        n116 = call "校准日志.vi"("table"="校准记录", "日志信息"=w203) -> ()  [unwired: 9 in, 1 out]
      }
      frame "Cal: Over" {
        n117 = global read "多参数全局变量.vi" "校准运行状态"() -> (w224:T7)
        n118 = Bundle By Name(cluster=w224, "DO"=FALSE) -> (w225:T7)
        n119 = global write "多参数全局变量.vi" "校准运行状态"(w225) -> ()
      }
      frame "idle", Default {
        n120 = event shown="[1] \"校准模式\": 值改变" {
          selector: _ -> [_ _ _ _ _ _ _ _ _]
          dyn-events: _ -> [_ _ _ _ _ _ _ _ _]
          timeout: 10 -> [_ _ _ _ _ _ _ _ _]
          tunnel: w237 -> [w240 w244 w249 w260 w269 w274 w283 w294 _]
          tunnel: [w239 w243 w250 w263 w273 w276 w287 w293 w296] -> w236
          tunnel: [w238 w241 w251 w262 w272 w275 w286 w291 w297] -> w235
          tunnel: w234 -> [w238 w241 w251 w262 w272 w275 w286 w291 w297]
          tunnel: w230 -> [_ _ _ _ w267 _ w281 _ _]
          event Timeout {
            n121 = event-data() -> ()  [unwired: 1 in, 3 out]
            n122 = call "Add State to Queue.vi"("State(s) In (\"\")"=w240) -> ("States Out"=w239:string)  [unwired: 14 in]
          }
          event "校准模式": Value Change {
            n123 = event-data() -> ()  [unwired: 1 in, 6 out]
            n124 = call "Add State to Queue.vi"("State(s) In (\"\")"=w244, "State(s) At Back (\"\")"="init: all\nidle" ("State(s) In (\"\")")) -> ("States Out"=w243:string)  [unwired: 13 in]
          }
          event "大气压力", "滤波设定": Mouse Down {
            n125 = event-data() -> ("CtlRef"=w248:refnum<vi>)  [unwired: 1 in, 7 out]
            n126 = property class="DigNum (严格)"(reference=w248) -> (reference out=w245:refnum<vi>, "Value"=w246:dbl)  [unwired: 1 in, 1 out]
            n127 = call "数字键盘.vi"("OldNumber"=w246) -> ("NewNumber"=w247:dbl)  [unwired: 1 in]
            n128 = property class="DigNum (严格)"(reference=w245, "Val(Sgnl)"=w247) -> ()  [unwired: 1 in, 2 out]
            n129 = call "Add State to Queue.vi"("State(s) In (\"\")"=w249) -> ("States Out"=w250:string)  [unwired: 14 in]
          }
          event "盐度": Mouse Down {
            n130 = event-data() -> ("CtlRef"=w261:refnum<vi>)  [unwired: 1 in, 7 out]
            n131 = global read "断电保存变量.vi" "Cond"() -> (w252:bool)
            n132 = case shown="真" w252 {
              tunnel: [_ w264] -> w257
              frame False {
              }
              frame True {
                n133 = Two Button Dialog(message="是否使用系统测试值自动补偿" ("消息")) -> (T button?=w264:bool)  [unwired: 2 in]
              }
            }
            n134 = global read "多参数全局变量.vi" "盐度显示"() -> (w256:T8)
            n135 = property class="DigNum (严格)"(reference=w261) -> (reference out=w258:refnum<vi>, "Value"=w254:sgl)  [unwired: 1 in, 1 out]
            n136 = Unbundle By Name(w256) -> ("测量值"=w255:sgl)
            n137 = Select(t=w255, s=w257, f=w254) -> (s? t:f=w253:sgl)
            n138 = call "数字键盘.vi"("OldNumber"=w253) -> ("NewNumber"=w259:dbl)  [unwired: 1 in]
            n139 = call "Add State to Queue.vi"("State(s) In (\"\")"=w260) -> ("States Out"=w263:string)  [unwired: 14 in]
            n140 = property class="DigNum (严格)"(reference=w258, "Val(Sgnl)"=w259) -> ()  [unwired: 1 in, 2 out]
          }
          event "大气压力": Value Change {
            n141 = event-data() -> ("NewVal"=w270:dbl)  [unwired: 1 in, 3 out]
            n142 = global read "多参数全局变量.vi" "MB session in"() -> (w271:refnum<class "MB_Master.lvclass">)
            n143 = call "纳清DO_大气压力写入.vi"("数值"=w270, "MB session in"=w271) -> ("error out"=w268:errorcluster)  [unwired: 8 in, 1 out]
            n144 = Enqueue Element At Opposite End(queue=w267, element=T1."DO" ("元素"), error in (no error)=w268) -> ()  [unwired: 1 in, 3 out]
            n145 = call "Add State to Queue.vi"("State(s) In (\"\")"=w269) -> ("States Out"=w273:string)  [unwired: 14 in]
          }
          event "滤波设定": Value Change {
            n146 = event-data() -> ()  [unwired: 1 in, 4 out]
            n147 = flat-sequence {
              frame #0 {
                n148 = global read "断电保存变量.vi" "滤波设置"() -> (w279:T4)
                n149 = local read "滤波设定"() -> (w277:dbl)
                n150 = Bundle By Name(cluster=w279, "DO"=w277) -> (w278:T4)
                n151 = global write "断电保存变量.vi" "滤波设置"(w278) -> ()
              }
              frame #1 {
                n152 = call "配置文件保存.vi"() -> ()  [unwired: 12 in]
              }
            }
            n153 = call "Add State to Queue.vi"("State(s) In (\"\")"=w274) -> ("States Out"=w276:string)  [unwired: 14 in]
          }
          event "盐度": Value Change {
            n154 = event-data() -> ("NewVal"=w284:sgl)  [unwired: 1 in, 5 out]
            n155 = global read "多参数全局变量.vi" "MB session in"() -> (w285:refnum<class "MB_Master.lvclass">)
            n156 = call "纳清DO_盐度写入.vi"("数值"=w284, "MB session in"=w285) -> ("error out"=w282:errorcluster)  [unwired: 8 in, 1 out]
            n157 = Enqueue Element At Opposite End(queue=w281, element=T1."DO" ("元素"), error in (no error)=w282) -> ()  [unwired: 1 in, 3 out]
            n158 = call "Add State to Queue.vi"("State(s) In (\"\")"=w283) -> ("States Out"=w287:string)  [unwired: 14 in]
          }
          event "校准启动": Value Change {
            n159 = event-data() -> ()  [unwired: 1 in, 6 out]
            n160 = global read "多参数全局变量.vi" "校准运行状态"() -> (w289:T7)
            n161 = call "Add State to Queue.vi"("State(s) In (\"\")"=w294, "State(s) At Back (\"\")"="init: all\nCal: Place standard solution\n Cal: Calibration process\nidle" ("State(s) In (\"\")")) -> ("States Out"=w293:string)  [unwired: 13 in]
            n162 = Bundle By Name(cluster=w289, "DO"=TRUE) -> (w290:T7)
            n163 = global write "多参数全局变量.vi" "校准运行状态"(w290) -> ()
          }
          event "校准停止": Value Change {
            n164 = event-data() -> ()  [unwired: 1 in, 6 out]
            n165 = call "Add State to Queue.vi"("State(s) In (\"\")"="init: all\nCal: Over\nidle" ("State(s) In (\"\")")) -> ("States Out"=w296:string)  [unwired: 14 in]
          }
        }
      }
    }
  }
